vi "Make CSRF Token.vi"(8 "error in (no error)":errorcluster, 10 "Token ID":string, 11 "Session In":refnum<class "Session.lvclass">) -> (0 "error out":errorcluster, 2 "Token":string, 3 "Session":refnum<class "Session.lvclass">)   [LabVIEW 2020, in "HTTP Server.lvlib"]
doc: "Sessions must be enabled.\n\nGenerates a string that should be integrated in a subsequent request to validate that the request isn't a replay attack. The specified ID and a random string are stored in the user's session to be validated against when that string is retrieved from the subsequent request. An example application for this CSRF token is to place it in a hidden field in a login form (or any form or POST request) so that it can be pulled from the form field once submitted and Validate CSRF Token.vi can be called with the returned token to ensure the request isn't spoofed or a replay from an expired session. For more details on CSRF, search for CSRF on OWASP."
uses:
  HTTP Server.lvlib
  Session/Session.lvclass
  lv-web-crypto/lv-crypto/Crypto/Crypto.lvlib
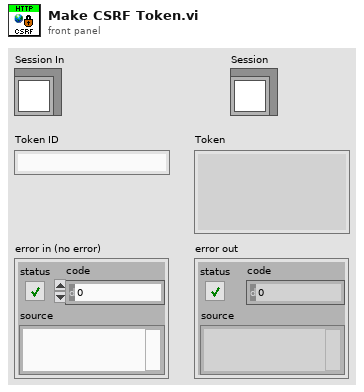
[diagram p1: front panel]
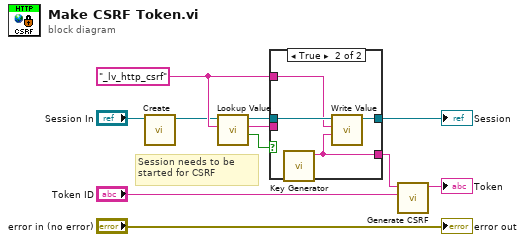
[diagram p0: block diagram]
diagram:
  w8 = "_lv_http_csrf" ("Name")
  # "Session needs to be started for CSRF"
  n1 = call "Create.vi"("Session in"="Session In") -> ("Session out"=w2:refnum<class "Session.lvclass">)  [unwired: 9 in, 1 out]
  n2 = call "Lookup Value.vi"("Name"=w8, "Session in"=w2) -> ("Not Found?"=w9:bool, "Value"=w10:string, "Session out"=w11:refnum<class "Session.lvclass">)  [unwired: 6 in, 1 out]
  n3 = case shown="True" w9 {
    tunnel: w11 -> [w13 w17]
    tunnel: w10 -> [w12 _]
    tunnel: w8 -> [_ w16]
    tunnel: [w13 w15] -> w7
    tunnel: [w12 w14] -> w5
    frame False {
    }
    frame True {
      n4 = call "Key Generator.vi"() -> ("Key"=w14:string)  [unwired: 10 in, 1 out]
      n5 = call "Write Value.vi"("Value"=w14, "Name"=w16, "Session in"=w17) -> ("Session out"=w15:refnum<class "Session.lvclass">)  [unwired: 6 in, 2 out]
    }
  }
  "Session" <- w7
  n6 = call "Generate CSRF.vi"("Token ID"="Token ID", "Key"=w5) -> ("Generated Token"=→"Token":string)  [unwired: 9 in]
  "error out" <- "error in (no error)"
